vi "Old VP.vi"(7 "Image Size":T1=enum."320x240") -> ()   [LabVIEW 2016]
doc: "This VI runs in parallel to other tasks. It gets images from the camera, processes them for color or shape and use that information to affect robot behavior."
uses:
  <vilib>/Rock Robotics/WPI/Camera/WPI_CameraWhite Balance Values.ctl
  <vilib>/Rock Robotics/WPI/Camera/WPI_CameraFrameRate.ctl
  <vilib>/Rock Robotics/WPI/Camera/WPI_CameraExposure Values.ctl
  <vilib>/Rock Robotics/Network Tables/NT Write Boolean.vi
  Robot Global Data.vi
  <vilib>/Rock Robotics/WPI/Camera/WPI_CameraImageSize.ctl
panel:
  in  "error in (no error)":errorcluster
  in  "Image Size Cam 2":T1=enum."320x240"
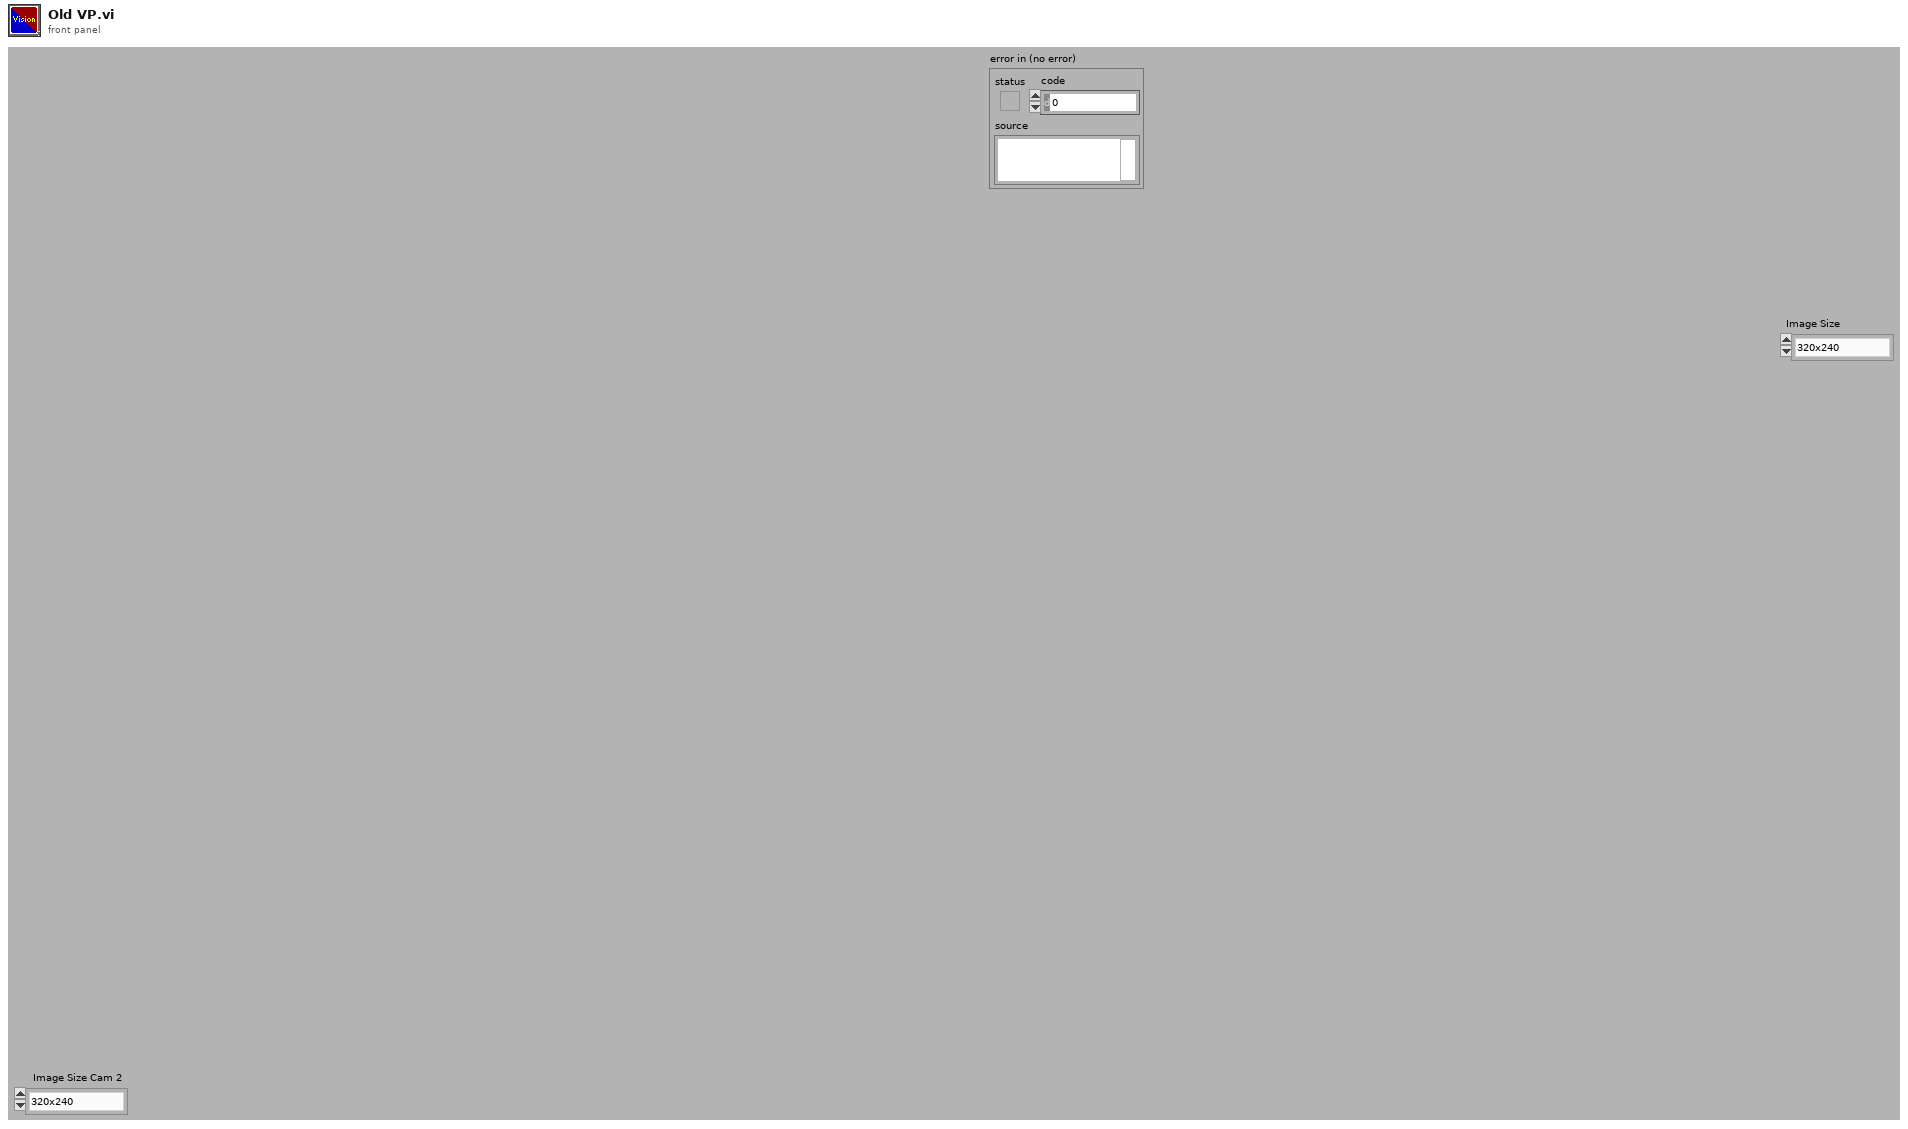
[diagram p1: front panel]
types:
  T1 = typedef "WPI_CameraImageSize.ctl" = enum16{"640x480", "320x240", "160x120", "Custom"}
  T2 = typedef "WPI_CameraExposure Values.ctl" = enum16{"Auto", "Flicker-free 50 Hz", "Flicker-free 60 Hz", "Hold current", "Custom"}
  T3 = typedef "WPI_CameraWhite Balance Values.ctl" = enum16{"Auto", "Fixed indoor", "Fixed outdoor 1", "Fixed outdoor 2", "Fixed fluorescent 1", "Fixed fluorescent 2", "Hold current", "Custom"}
  T4 = typedef "WPI_CameraFrameRate.ctl" = u32
  T5 = typedef "Image Type" = u32
  T6 = typedef "WPI_CameraDevRef.ctl" = cluster{"Camera Address":string, "CameraStatus":errorcluster}
  T7 = typedef "IMAQ Image.ctl" = refnum<image>
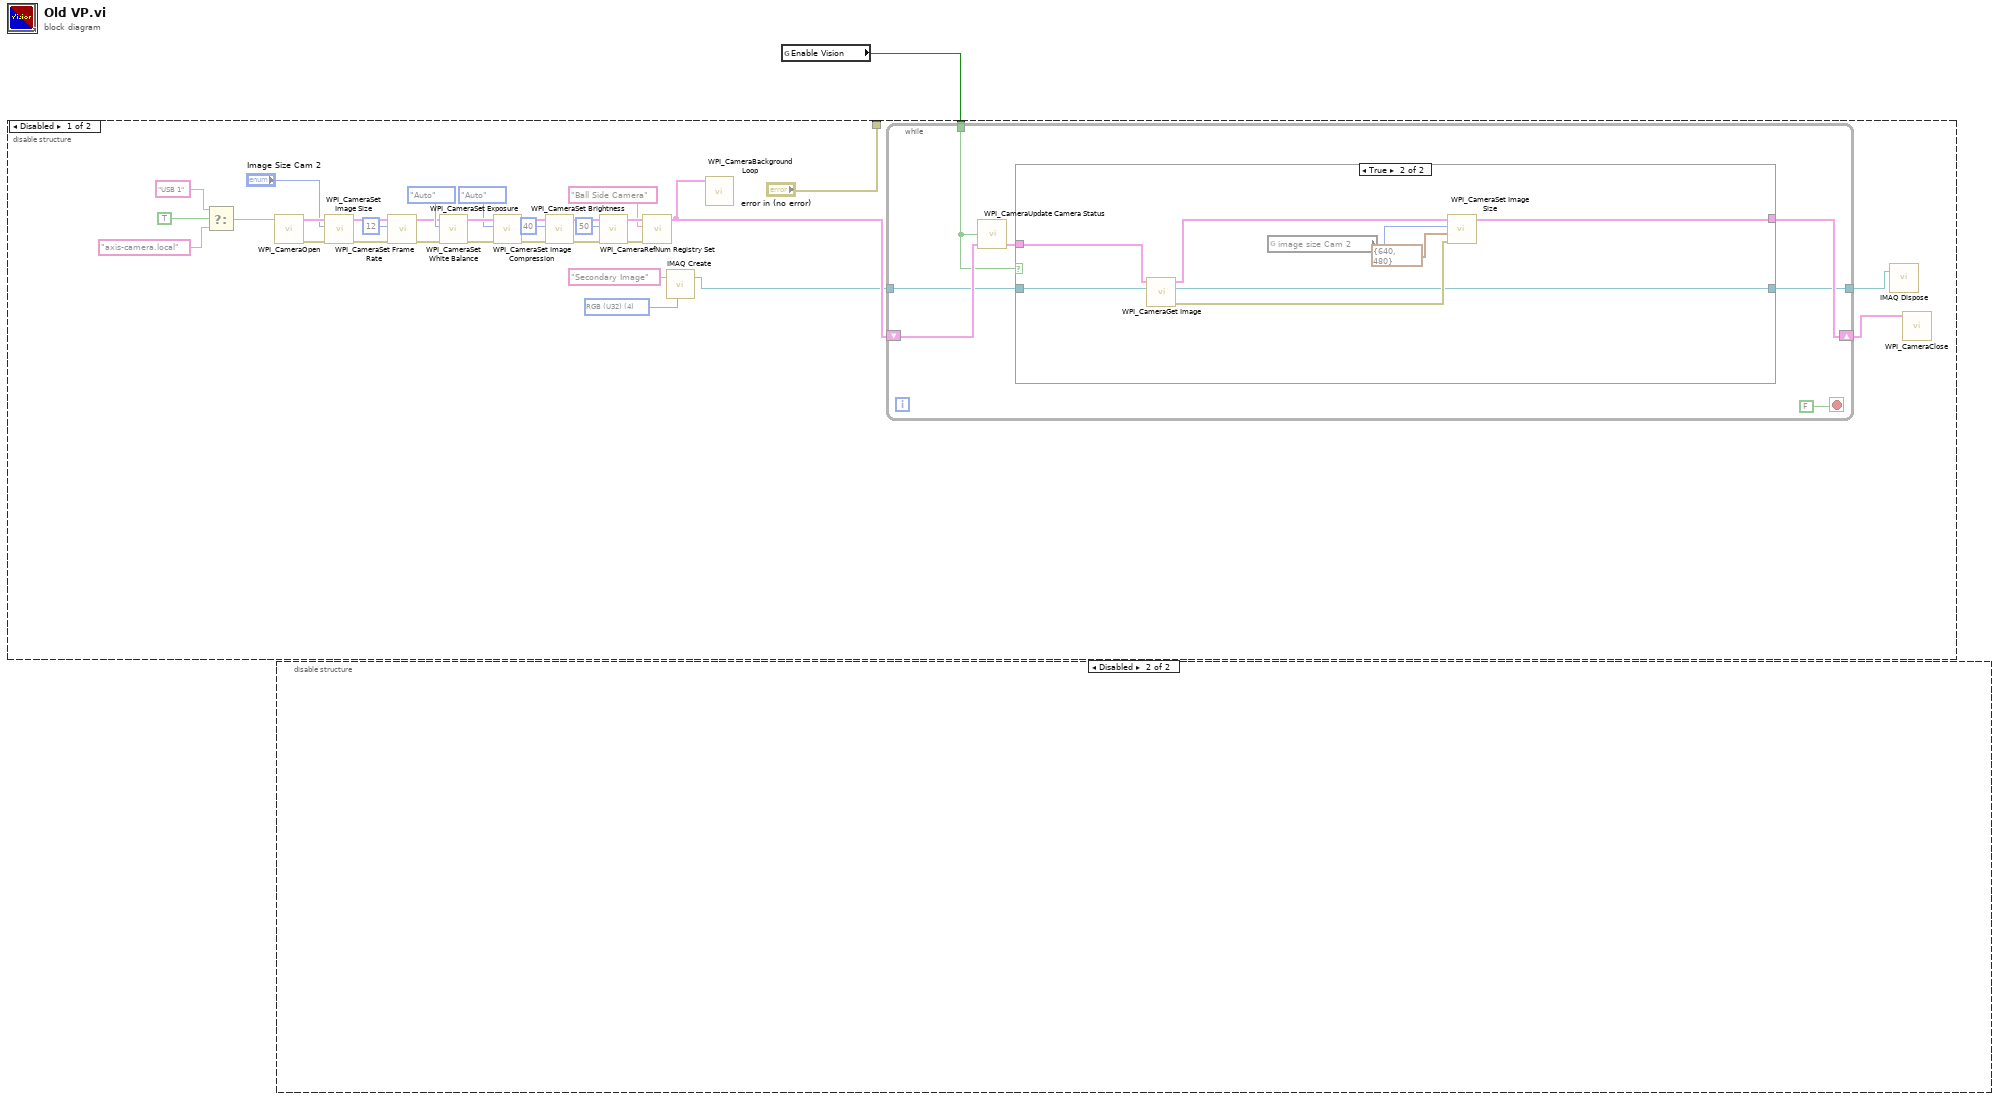
[diagram p0: block diagram]
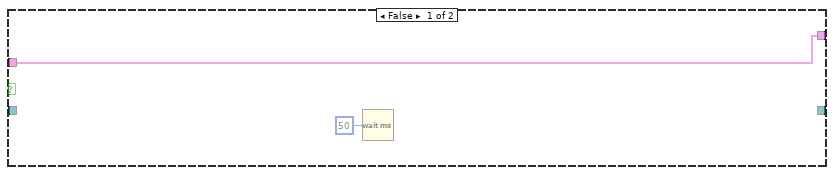
[diagram p2: hidden frame]
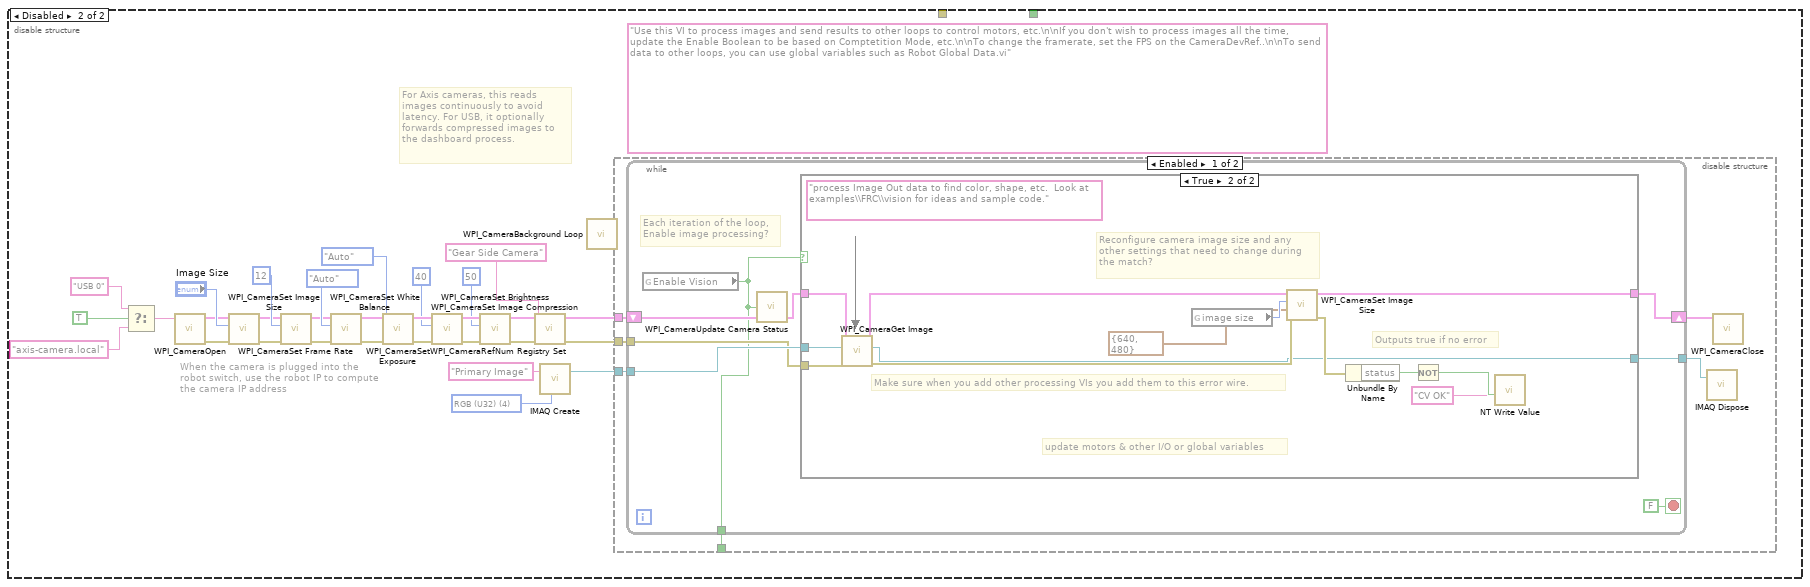
[diagram p3: hidden frame]
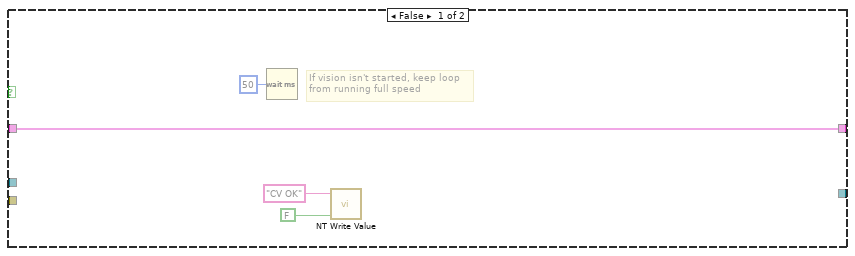
[diagram p4: hidden frame]
diagram:
  n1 = disable-structure shown="Disabled" {
    frame Enabled {
    }
    frame Disabled {
    }
  }
  n2 = global read "Robot Global Data.vi" "Enable Vision"() -> (w1:bool)
  n3 = disable-structure shown="Disabled" {
    disable-tunnel: ["error in (no error)" _] -> _
    disable-tunnel: w1 -> [w4 _]
    frame Disabled {
      w8 = T5 4 items=["Grayscale (U8)", "Grayscale (I16)", "Grayscale (SGL)", "Complex (CSG)", "RGB (U32)", "HSL (U32)", "RGB (U64)"] ("Image Type")
      n4 = Select(t="USB 1" ("format string"), s=TRUE ("dot notation? (F)"), f="axis-camera.local" ("format string")) -> (s? t:f=w30:string)
      n5 = call <vilib>:"WPI_CameraOpen.vi"("Camera Address"=w30) -> ("error out"=w16:errorcluster, "CameraDevRef"=w28:T6)  [unwired: 1 in, 8 out]
      n6 = call <vilib>:"WPI_CameraSet Image Size.vi"("error in (no error)"=w16, "Image Size"="Image Size Cam 2", "CameraDevRef"=w28) -> ("error out"=w15:errorcluster, "CameraDevRef Out"=w29:T6)  [unwired: 1 in, 6 out]
      n7 = call <vilib>:"WPI_CameraSet Frame Rate.vi"("error in (no error)"=w15, "Frame Rate (fps)"=T4 12, "CameraDevRef"=w29) -> ("error out"=w14:errorcluster, "CameraDevRef Out"=w25:T6)  [unwired: 7 out]
      n8 = call <vilib>:"WPI_CameraSet White Balance.vi"("error in (no error)"=w14, "White Balance"=WPI_CameraWhite_Balance_Values."Auto", "CameraDevRef"=w25) -> ("error out"=w13:errorcluster, "CameraDevRef Out"=w24:T6)  [unwired: 1 in, 6 out]
      n9 = call <vilib>:"WPI_CameraSet Exposure.vi"("error in (no error)"=w13, "Exposure"=WPI_CameraExposure_Values."Auto", "CameraDevRef"=w24) -> ("error out"=w12:errorcluster, "CameraDevRef Out"=w22:T6)  [unwired: 1 in, 6 out]
      n10 = call <vilib>:"WPI_CameraSet Image Compression.vi"("error in (no error)"=w12, "Compression"=40, "CameraDevRef"=w22) -> ("error out"=w11:errorcluster, "CameraDevRef Out"=w20:T6)  [unwired: 7 out]
      n11 = call <vilib>:"WPI_CameraSet Brightness.vi"("error in (no error)"=w11, "Brightness"=50, "CameraDevRef"=w20) -> ("error out"=w10:errorcluster, "CameraDevRef Out"=w18:T6)  [unwired: 7 out]
      n12 = call <vilib>:"WPI_CameraRefNum Registry Set.vi"("error in (no error)"=w10, "refnum name"="Ball Side Camera", "CameraDevRef"=w18) -> ("CameraDevRef"=w6:T6)  [unwired: 1 in, 7 out]
      n13 = call "IMAQ Create"("Image Name"="Secondary Image", "Image Type"=w8) -> ("New Image"=w5:T7)  [unwired: 2 in, 2 out]
      n14 = call <vilib>:"WPI_CameraBackground Loop.vi"("CameraDevRef"=w6) -> ()  [unwired: 11 in]
      n15 = while {
        shift-right: [w36] -> w3
        shift-left: w6 -> [w40]
        tunnel: w4 -> [w39]
        tunnel: w5 -> [w37]
        tunnel: [w35] -> w2
        stop <- FALSE stop-if-true
        n16 = call <vilib>:"WPI_CameraUpdate Camera Status.vi"("CameraDevRef In"=w40, "Enable Vision"=w39) -> ("CameraDevRef Out"=w41:T6)  [unwired: 3 in]
        n17 = case shown="True" w39 {
          tunnel: [w42 w50] -> w36
          tunnel: w41 -> [w42 w49]
          tunnel: w37 -> [_ w46]
          tunnel: [_ w44] -> w35
          frame False {
            n18 = Wait (ms)(milliseconds to wait=u32 50) -> ()  [unwired: 1 out]
          }
          frame True {
            n19 = call <vilib>:"WPI_CameraGet Image.vi"("Image"=w46, "CameraDevRef"=w49) -> ("error out"=w51:errorcluster, "Image Out"=w44:T7, "CameraDevRef Out"=w48:T6)  [unwired: 1 in, 6 out]
            n20 = global read "Robot Global Data.vi" "image size Cam 2"() -> (w47:T1)
            n21 = call <vilib>:"WPI_CameraSet Image Size.vi"("error in (no error)"=w51, "Size W,H (pix)"=cluster{i32, i32} {640, 480}, "Image Size"=w47, "CameraDevRef"=w48) -> ("CameraDevRef Out"=w50:T6)  [unwired: 7 out]
          }
        }
      }
      n22 = call "IMAQ Dispose"("Image"=w2) -> ()  [unwired: 5 in, 1 out]
      n23 = call <vilib>:"WPI_CameraClose.vi"("CameraDevRef"=w3) -> ()  [unwired: 1 in, 10 out]
    }
    frame Disabled {
      (unwired) "Use this VI to process images and send results to other loops to control motors, etc.\n\nIf you don't wish to process images all the time, update the Enable Boolean to be based on Comptetition Mode, etc.\n\nTo change the framerate, set the FPS on the CameraDevRef..\n\nTo send data to other loops, you can use global variables such as Robot Global Data.vi"
      w52 = T5 4 items=["Grayscale (U8)", "Grayscale (I16)", "Grayscale (SGL)", "Complex (CSG)", "RGB (U32)", "HSL (U32)", "RGB (U64)"] ("Image Type")
      # "When the camera is plugged into the\nrobot switch, use the robot IP to compute\nthe camera IP address"
      # "For Axis cameras, this reads\nimages continuously to avoid\nlatency. For USB, it optionally\nforwards compressed images to\nthe dashboard process."
      n24 = Select(t="USB 0" ("format string"), s=TRUE ("dot notation? (F)"), f="axis-camera.local" ("format string")) -> (s? t:f=w78:string)
      n25 = call <vilib>:"WPI_CameraOpen.vi"("Camera Address"=w78) -> ("error out"=w64:errorcluster, "CameraDevRef"=w63:T6)  [unwired: 1 in, 8 out]
      n26 = call <vilib>:"WPI_CameraSet Image Size.vi"("error in (no error)"=w64, "Image Size"="Image Size", "CameraDevRef"=w63) -> ("error out"=w65:errorcluster, "CameraDevRef Out"=w62:T6)  [unwired: 1 in, 6 out]
      n27 = call <vilib>:"WPI_CameraSet Frame Rate.vi"("error in (no error)"=w65, "Frame Rate (fps)"=T4 12, "CameraDevRef"=w62) -> ("error out"=w66:errorcluster, "CameraDevRef Out"=w60:T6)  [unwired: 7 out]
      n28 = call <vilib>:"WPI_CameraSet White Balance.vi"("error in (no error)"=w66, "White Balance"=WPI_CameraWhite_Balance_Values."Auto", "CameraDevRef"=w60) -> ("error out"=w67:errorcluster, "CameraDevRef Out"=w61:T6)  [unwired: 1 in, 6 out]
      n29 = call <vilib>:"WPI_CameraSet Exposure.vi"("error in (no error)"=w67, "Exposure"=WPI_CameraExposure_Values."Auto", "CameraDevRef"=w61) -> ("error out"=w68:errorcluster, "CameraDevRef Out"=w58:T6)  [unwired: 1 in, 6 out]
      n30 = call <vilib>:"WPI_CameraSet Image Compression.vi"("error in (no error)"=w68, "Compression"=40, "CameraDevRef"=w58) -> ("error out"=w69:errorcluster, "CameraDevRef Out"=w59:T6)  [unwired: 7 out]
      n31 = call <vilib>:"WPI_CameraSet Brightness.vi"("error in (no error)"=w69, "Brightness"=50, "CameraDevRef"=w59) -> ("error out"=w71:errorcluster, "CameraDevRef Out"=w70:T6)  [unwired: 7 out]
      n32 = call <vilib>:"WPI_CameraRefNum Registry Set.vi"("error in (no error)"=w71, "refnum name"="Gear Side Camera", "CameraDevRef"=w70) -> ("error out"=w80:errorcluster, "CameraDevRef"=w74:T6)  [unwired: 1 in, 6 out]
      n33 = call "IMAQ Create"("Image Name"="Primary Image", "Image Type"=w52) -> ("New Image"=w54:T7)  [unwired: 2 in, 2 out]
      n34 = disable-structure shown="Enabled" {
        disable-tunnel: w54 -> [w87 _]
        disable-tunnel: w74 -> [w86 _]
        disable-tunnel: w80 -> [w85 _]
        disable-tunnel: [w82 _] -> _
        frame Enabled {
          n35 = call <vilib>:"WPI_CameraBackground Loop.vi"("CameraDevRef"=w86) -> ()  [unwired: 11 in]
          n36 = while {
            shift-right: [w94] -> w84
            shift-left: w86 -> [w92]
            tunnel: w87 -> [w93]
            tunnel: w85 -> [w90]
            tunnel: [w89] -> w82
            tunnel: [w88] -> w83
            stop <- FALSE stop-if-true
            # "Each iteration of the loop,\nEnable image processing?"
            n37 = global read "Robot Global Data.vi" "Enable Vision"() -> (w89:bool)
            n38 = call <vilib>:"WPI_CameraUpdate Camera Status.vi"("CameraDevRef In"=w92, "Enable Vision"=w89) -> ("CameraDevRef Out"=w91:T6)  [unwired: 3 in]
            n39 = case shown="True" w89 {
              tunnel: w93 -> [_ w111]
              tunnel: [w99 w112] -> w94
              tunnel: w91 -> [w99 w109]
              tunnel: w90 -> [_ w107]
              tunnel: [_ w100] -> w88
              frame False {
                # "If vision isn't started, keep loop\nfrom running full speed"
                n40 = Wait (ms)(milliseconds to wait=u32 50) -> ()  [unwired: 1 out]
                n41 = call-poly <vilib>:"NT Write Value.vi"("Boolean"=FALSE, "Name"="CV OK") -> ()  [unwired: 9 in, 1 out]
              }
              frame True {
                (unwired) "process Image Out data to find color, shape, etc.  Look at examples\\FRC\\vision for ideas and sample code."
                # "Outputs true if no error"
                # "Make sure when you add other processing VIs you add them to this error wire."
                # "update motors & other I/O or global variables"
                # "Reconfigure camera image size and any\nother settings that need to change during\nthe match?"
                n42 = call <vilib>:"WPI_CameraGet Image.vi"("error in (no error)"=w107, "Image"=w111, "CameraDevRef"=w109) -> ("error out"=w106:errorcluster, "Image Out"=w100:T7, "CameraDevRef Out"=w108:T6)  [unwired: 6 out]
                n43 = global read "Robot Global Data.vi" "image size"() -> (w110:T1)
                n44 = call <vilib>:"WPI_CameraSet Image Size.vi"("error in (no error)"=w106, "Size W,H (pix)"=cluster{i32, i32} {640, 480}, "Image Size"=w110, "CameraDevRef"=w108) -> ("error out"=w104:errorcluster, "CameraDevRef Out"=w112:T6)  [unwired: 6 out]
                n45 = Unbundle By Name(w104) -> ("status"=w105:bool)
                n46 = Not(x=w105) -> (.not. x?=w103:bool)
                n47 = call-poly <vilib>:"NT Write Value.vi"("Boolean"=w103, "Name"="CV OK") -> ()  [unwired: 9 in, 1 out]
              }
            }
          }
          n48 = call "IMAQ Dispose"("Image"=w83) -> ()  [unwired: 5 in, 1 out]
          n49 = call <vilib>:"WPI_CameraClose.vi"("CameraDevRef"=w84) -> ()  [unwired: 1 in, 10 out]
        }
        frame Disabled {
        }
      }
    }
  }
